vi "PSLDAQ_AcquireStop.vi"(1 "Trigger":bool, 2 "Handle In":T1) -> ()   [LabVIEW 2010]
doc: "1. 설명\n a. 통신 연결된 PSL- DAQ 장치로부터 데이터 획득 중지\n\n2. 기능\n a. 통신 연결된 PSL-DAQ 장치로 데이터 획득 중지 명령을 보냄 \n \n3. 터미널\n a. 터미널 입력\n ○ Handle In : 장치 핸들 \n ○ Trigger : PSLDAQ_AcquireStop VI를 1회만 동작시키기 위한 트리거 신호\n\n4. 주의\n a. PSL-DAQ 장치와 통신 연결된 경우에 정상적으로 동작함.\n b. Trigger 입력으로 Boolean형 컨트롤을 사용하는 경우 1회만 입력 가능하도록 컨트롤 속성을\n 수정하여야 함.\n ㆍ“컨트롤 속성>동작>놓을 때 래치” 로 설정(영문인 경우 Latch When Release)하면 버튼을 \n 클릭한 경우 1회만 Trigger 값이 발생함."
uses:
  PSLDAQ_Dll.dll
panel:
  # "PSLDAQ_AcquireStop\n\n1. 설명\n  a. 통신 연결된 PSL- DAQ 장치로부터 데이터 획득 중지\n\n2. 기능\n  a. 통신 연결된 PSL-DAQ 장치로 데이터 획득 중지 명령을 보냄 \n      \n3. 터미널\n   a. 터미널 입력\n    ○ Handle In : 장치 핸들 \n    ○ Trigger : PSLDAQ_AcquireStop VI를 1회만 동작시키기 위한 트리거 신호\n\n4. 주의\n  a. PSL-DAQ 장치와 통신 연결된 경우에 정상적으로 동작함.\n  b. Trigger 입력으로 Boolean형 컨트롤을 사용하는 경우 1회만 입력 가능하도록 컨트롤 속성을\n      수정하여야 함.\n      ㆍ“컨트롤 속성>동작>놓을 때 래치” 로 설정(영문인 경우 Latch When Release)하면 버튼을 \n          클릭한 경우 1회만 Trigger 값이 발생함."
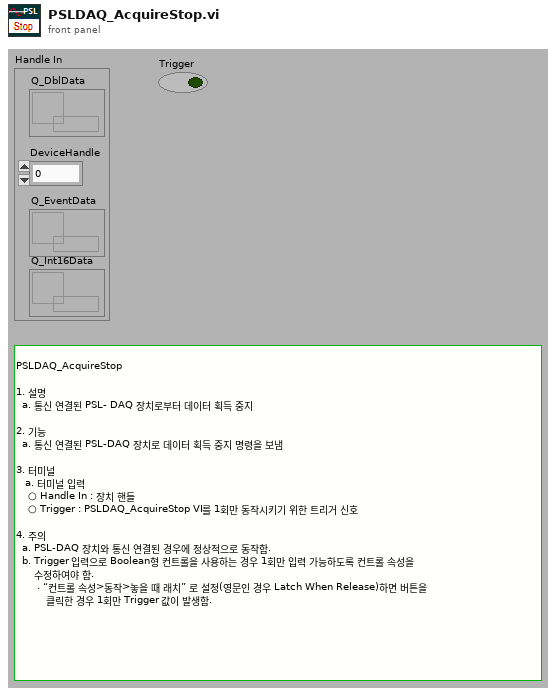
[diagram p1: front panel]
types:
  T1 = cluster{"Q_DblData":refnum<queue>, "DeviceHandle":u32, "Q_EventData":refnum<queue>, "Q_Int16Data":refnum<queue>}
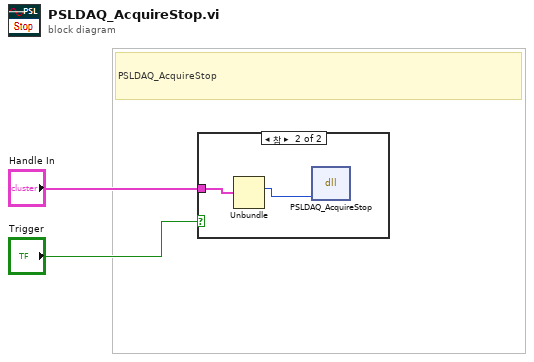
[diagram p0: block diagram]
diagram:
  # "PSLDAQ_AcquireStop"
  n1 = case shown="참" "Trigger" {
    tunnel: "Handle In" -> [_ w3]
    frame False {
    }
    frame True {
      n2 = Unbundle(w3) -> ("DeviceHandle"=w4:u32)  [unwired: 3 out]
      n3 = dll-call lib="D:/PSL-DAQ LabVIEW Library/PSLDAQ_Dll.dll" fn="PSLDAQ_AcquireStop"("DeviceHandle"=w4) -> ()  [unwired: 5 in, 2 out]
    }
  }
